vi "TLE.vi"(2 "TLE - Enter the two last lines - verify that the TLE is up to date":string) -> (12 "number of minutes \nof the epoch (min)":i32, 13 "n0 Mean movement (revolutions per day)":dbl format="%#_13g", 14 "B* Balistic coefficient":dbl format="%#_13g", 15 "i0 Orbit inclinaison\nregarding the earth equator (°)":dbl format="%#_13g", 16 "Ohm0 Right ascension of the\norbit ascending node (°)":dbl format="%#_13g", 17 "e0 Excentricity":dbl format="%#_13g", 18 "omega0 Perigee argument (°)":dbl format="%#_13g", 19 "M0 Mean anomaly (°)":dbl format="%#_13g")   [LabVIEW 2014]
panel:
  out "number of minutes since\nthe epoch (t-t0) (min)":dbl format="%#_13g"
  out "number of seconds between \nJanuary 1st 1904 and January 1st 2015":dbl format="%#_13g"
  out "number of seconds since the \nJanuary 1st 1904":dbl format="%#_13g"
  out "fraction of the day":dbl format="%#_13g"
  out "number of the day during the \nyear where the TLE has been determined":dbl format="%#_13g"
  out "Checksum (modulo 10)":dbl format="%#_13g"
  out "Number of revolutions when these\n\nelements have been determined":dbl format="%#_13g"
  out "Number US Space Command":dbl format="%#_13g"
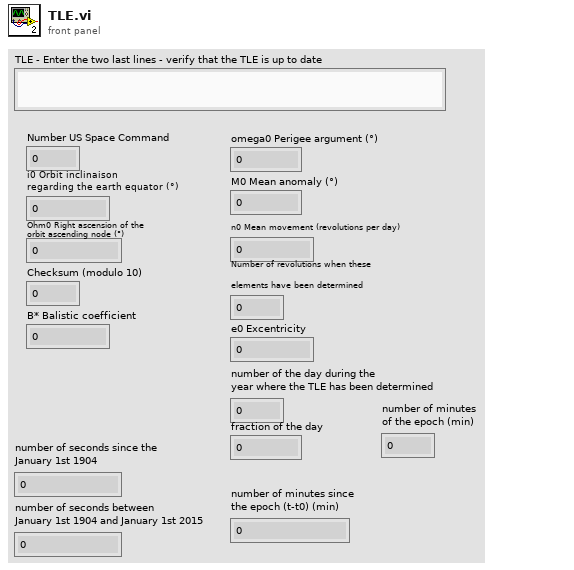
[diagram p1: front panel]
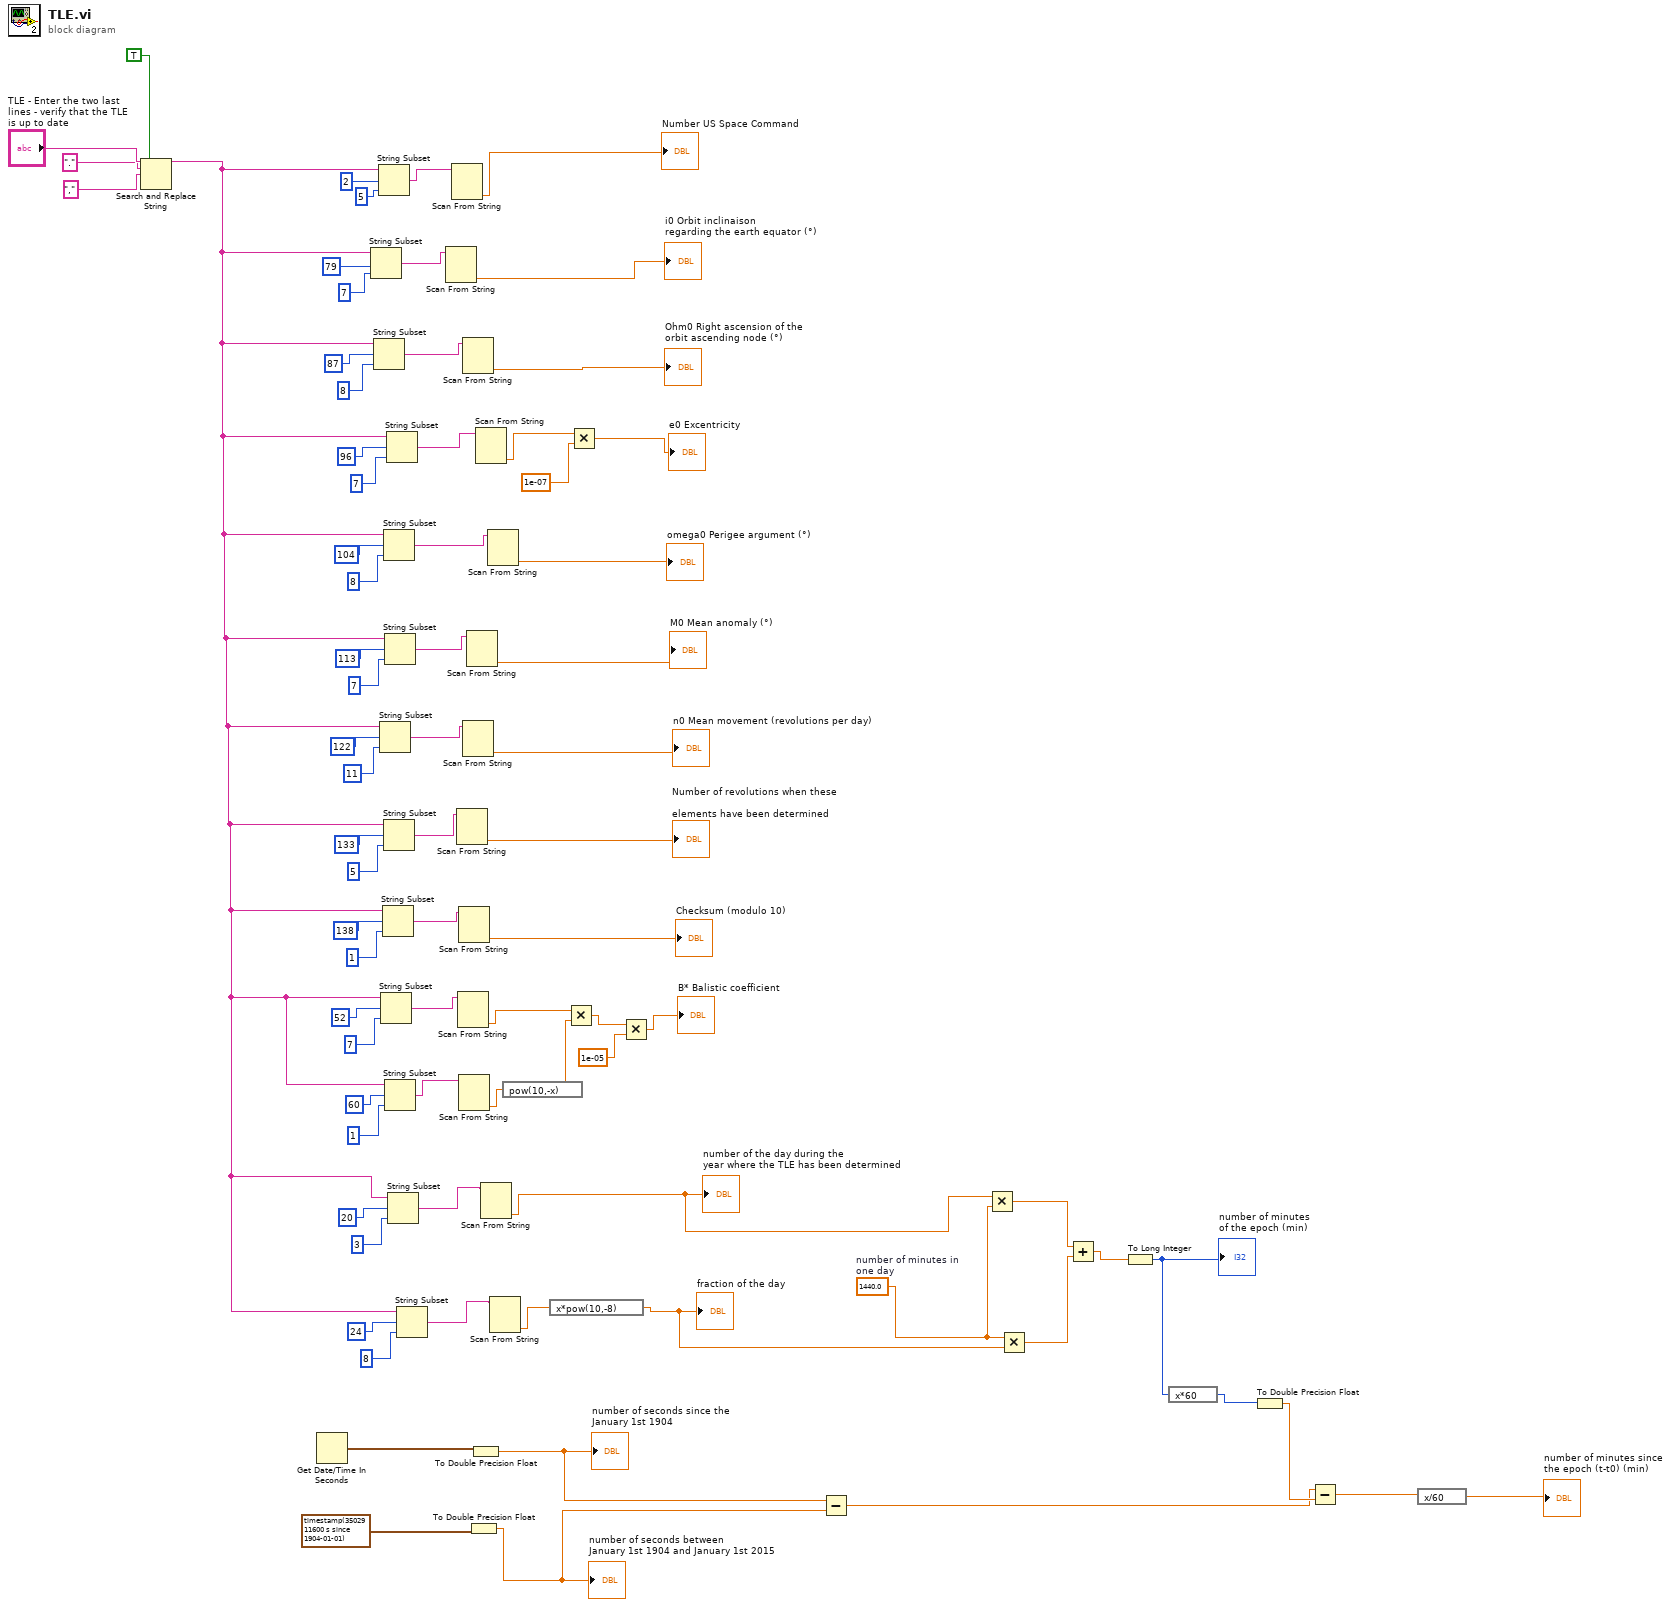
[diagram p0: block diagram]
diagram:
  w15 = 1440.0  # number of minutes in one day
  n1 = Search and Replace String(replace all?=TRUE, input string="TLE - Enter the two last lines - verify that the TLE is up to date", search string=".", replace string=",") -> (result string=w18:string)  [unwired: 4 in, 3 out]
  n2 = Get Date/Time In Seconds() -> (seconds since 1Jan1904=w10:timestamp)
  n3 = String Subset(string=w18, offset (0)=79, length (rest)=7) -> (substring=w56:string)
  n4 = String Subset(string=w18, offset (0)=87, length (rest)=8) -> (substring=w54:string)
  n5 = String Subset(string=w18, offset (0)=2, length (rest)=5) -> (substring=w58:string)
  n6 = String Subset(string=w18, offset (0)=122, length (rest)=11) -> (substring=w47:string)
  n7 = String Subset(string=w18, offset (0)=52, length (rest)=7) -> (substring=w34:string)
  n8 = String Subset(string=w18, offset (0)=138, length (rest)=1) -> (substring=w43:string)
  n9 = String Subset(string=w18, offset (0)=104, length (rest)=8) -> (substring=w51:string)
  n10 = String Subset(string=w18, offset (0)=133, length (rest)=5) -> (substring=w45:string)
  n11 = String Subset(string=w18, offset (0)=113, length (rest)=7) -> (substring=w49:string)
  n12 = String Subset(string=w18, offset (0)=60, length (rest)=1) -> (substring=w33:string)
  n13 = String Subset(string=w18, offset (0)=96, length (rest)=7) -> (substring=w52:string)
  n14 = String Subset(string=w18, offset (0)=20, length (rest)=3) -> (substring=w22:string)
  n15 = String Subset(string=w18, offset (0)=24, length (rest)=8) -> (substring=w19:string)
  n16 = Scan From String(input string=w56) -> (output 1=→"i0 Orbit inclinaison\nregarding the earth equator (°)":dbl)  [unwired: 4 in, 3 out]
  n17 = Scan From String(input string=w58) -> (output 1=→"Number US Space Command":dbl)  [unwired: 4 in, 3 out]
  n18 = Scan From String(input string=w45) -> (output 1=→"Number of revolutions when these\n\nelements have been determined":dbl)  [unwired: 4 in, 3 out]
  n19 = Scan From String(input string=w34) -> (output 1=w28:dbl)  [unwired: 4 in, 3 out]
  n20 = Scan From String(input string=w43) -> (output 1=→"Checksum (modulo 10)":dbl)  [unwired: 4 in, 3 out]
  n21 = Scan From String(input string=w33) -> (output 1=w30:dbl)  [unwired: 4 in, 3 out]
  n22 = Scan From String(input string=w54) -> (output 1=→"Ohm0 Right ascension of the\norbit ascending node (°)":dbl)  [unwired: 4 in, 3 out]
  n23 = Scan From String(input string=w47) -> (output 1=→"n0 Mean movement (revolutions per day)":dbl)  [unwired: 4 in, 3 out]
  n24 = Scan From String(input string=w49) -> (output 1=→"M0 Mean anomaly (°)":dbl)  [unwired: 4 in, 3 out]
  n25 = To Double Precision Float(number=timestamp(3502911600 s since 1904-01-01)) -> (double precision float=w7:dbl)
  "number of seconds between \nJanuary 1st 1904 and January 1st 2015" <- w7
  n26 = To Double Precision Float(number=w10) -> (double precision float=w6:dbl)
  "number of seconds since the \nJanuary 1st 1904" <- w6
  n27 = Scan From String(input string=w52) -> (output 1=w37:dbl)  [unwired: 4 in, 3 out]
  n28 = Scan From String(input string=w22) -> (output 1=w14:dbl)  [unwired: 4 in, 3 out]
  "number of the day during the \nyear where the TLE has been determined" <- w14
  n29 = Scan From String(input string=w51) -> (output 1=→"omega0 Perigee argument (°)":dbl)  [unwired: 4 in, 3 out]
  n30 = Scan From String(input string=w19) -> (output 1=w17:dbl)  [unwired: 4 in, 3 out]
  n31 = expression code="pow(10,-x)"(w30) -> (w29:dbl)
  n32 = expression code="x*pow(10,-8)"(w17) -> (w16:dbl)
  "fraction of the day" <- w16
  n33 = Multiply(x=w28, y=w29) -> (x*y=w27:dbl)
  n34 = Multiply(x=w37, y=1e-07) -> (x*y=→"e0 Excentricity":dbl)
  n35 = Multiply(x=w27, y=1e-05) -> (x*y=→"B* Balistic coefficient":dbl)
  n36 = Subtract(x=w6, y=w7) -> (x-y=w4:dbl)
  n37 = Multiply(x=w14, y=w15) -> (x*y=w13:dbl)
  n38 = Multiply(x=w15, y=w16) -> (x*y=w12:dbl)
  n39 = Add(x=w13, y=w12) -> (x+y=w11:dbl)
  n40 = To Long Integer(number=w11) -> (32bit integer=w8:i32)
  "number of minutes \nof the epoch (min)" <- w8
  n41 = expression code="x*60"(w8) -> (w1:i32)
  n42 = To Double Precision Float(number=w1) -> (double precision float=w5:dbl)
  n43 = Subtract(x=w4, y=w5) -> (x-y=w3:dbl)
  n44 = expression code="x/60"(w3) -> (→"number of minutes since\nthe epoch (t-t0) (min)":dbl)
